vi "FM Get Info.vi"() -> (0 "Offset (V)":dbl format="%.1f", 1 "Amplitude (V)":dbl format="%.1f")   [LabVIEW 2009]
uses:
  MWC Global.vi
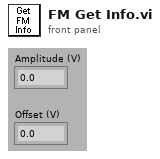
[diagram p1: front panel]
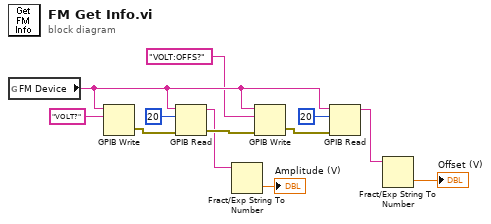
[diagram p0: block diagram]
diagram:
  n1 = global read "MWC Global.vi" "FM Device"() -> (w4:string)
  n2 = GPIB Write(0:w4, 1:"VOLT?" ("data")) -> (6:w11:errorcluster)  [unwired: 3 in, 1 out]
  n3 = GPIB Read(0:w4, 1:20 ("byte count"), 3:w11) -> (5:w8:string, 7:w9:errorcluster)  [unwired: 2 in, 1 out]
  n4 = Fract/Exp String To Number(string=w8) -> (number=→"Amplitude (V)":dbl)  [unwired: 3 in, 1 out]
  n5 = GPIB Write(0:w4, 1:"VOLT:OFFS?" ("data"), 3:w9) -> (6:w10:errorcluster)  [unwired: 2 in, 1 out]
  n6 = GPIB Read(0:w4, 1:20 ("byte count"), 3:w10) -> (5:w6:string)  [unwired: 2 in, 2 out]
  n7 = Fract/Exp String To Number(string=w6) -> (number=→"Offset (V)":dbl)  [unwired: 3 in, 1 out]
